vi "Find Worker Items.vi"(11 "Item Ref In":T1) -> (1 "Is Worker?":bool, 2 "Worker Items":T2, 3 "Item Ref":T1)   [LabVIEW 2020, in "FlexWorker_Provider.lvlib"]
uses:
  FlexWorker_Provider.lvlib
  <resource>/Framework/Providers/API/ItemRef.ctl
  Worker Items.ctl
  Worker Item.ctl
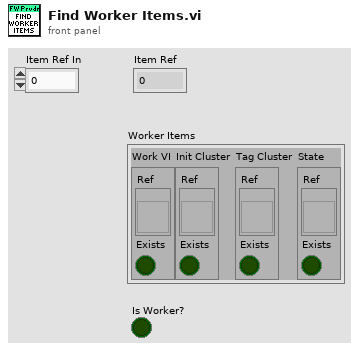
[diagram p1: front panel]
types:
  T1 = typedef "ItemRef.ctl" = u64
  T2 = typedef "FlexWorker_Provider.lvlib/Worker Items.ctl" = cluster{"Work VI":T3, "Init Cluster":T3, "Tag Cluster":T3, "State":T3}
  T3 = typedef "FlexWorker_Provider.lvlib/Worker Item.ctl" = cluster{"Ref":refnum<vi>, "Exists":bool}
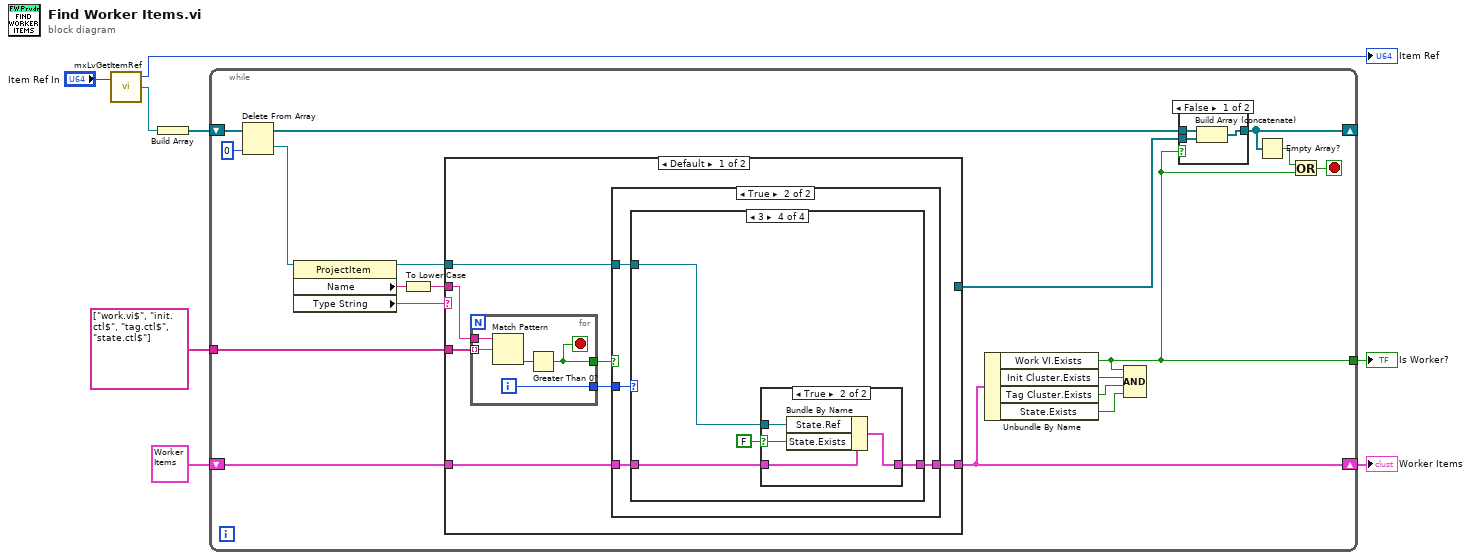
[diagram p0: block diagram]
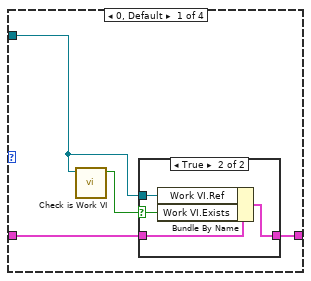
[diagram p4: hidden frame]
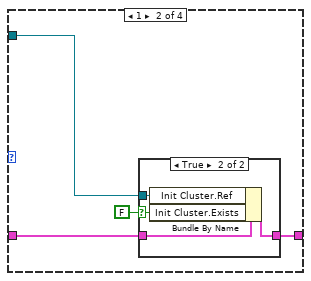
[diagram p6: hidden frame]
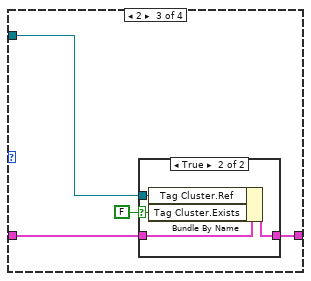
[diagram p8: hidden frame]
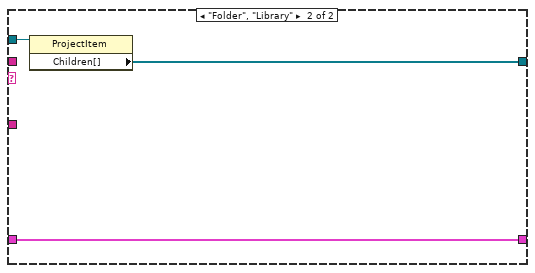
[diagram p11: hidden frame]
diagram:
  n1 = call <resource>:"mxLvGetItemRef.vi"("Item"="Item Ref In") -> ("Item"=→"Item Ref":T1, "Item Refnum"=w8:refnum<vi>)  [unwired: 1 in, 1 out]
  n2 = Build Array(w8) -> (w6:refnum<vi>[])
  n3 = while {
    shift-right: [w18] -> _
    shift-left: w6 -> [w27]
    shift-right: [w10] -> w4
    shift-left: T2 {"Work VI"={"Ref"=refnum, "Exists"=FALSE}, "Init Cluster"={"Ref"=refnum, "Exists"=FALSE}, "Tag Cluster"={"Ref"=refnum, "Exists"=FALSE}, "State"={"Ref"=refnum, "Exists"=FALSE}} ("Worker Items") -> [w20]
    tunnel: [w9] -> w3
    tunnel: string[] ["work.vi$", "init.ctl$", "tag.ctl$", "state.ctl$"] -> [w11]
    stop <- w15 stop-if-true
    n4 = Delete From Array(array=w27, index=0) -> (deleted portion=w25:refnum<vi>, array with subset deleted=w17:refnum<vi>[])  [unwired: 1 in]
    n5 = property class="ProjectItem"(reference=w25) -> (reference out=w23:refnum<vi>, "Name"=w24:string, "Type String"=w21:string)  [unwired: 1 in, 1 out]
    n6 = To Lower Case(string=w24) -> (all lower case string=w22:string)
    n7 = case shown="Default" w21 {
      tunnel: w23 -> [w34 w87]
      tunnel: w22 -> [w38 _]
      tunnel: w20 -> [w33 w85]
      tunnel: [_ w86] -> w16
      tunnel: [w32 w85] -> w10
      tunnel: w11 -> [w37 _]
      frame Default {
        n8 = for {
          tunnel: w38 -> [w84]
          tunnel: w37 -> [w83] mode=indexing
          tunnel: [w82] -> w35
          tunnel: [w80] -> w36
          i -> [w82]
          stop <- w80 stop-if-true
          n9 = Match Pattern(string=w84, regular expression=w83) -> (offset past match=w81:i32)  [unwired: 1 in, 3 out]
          n10 = Greater Than 0?(x=w81) -> (x > 0?=w80:bool)
        }
        n11 = case shown="True" w36 {
          tunnel: w35 -> [_ w42]
          tunnel: w34 -> [_ w43]
          tunnel: w33 -> [w39 w41]
          tunnel: [w39 w40] -> w32
          frame False {
            # "Not an item of interest"
          }
          frame True {
            n12 = case shown="3" w42 {
              tunnel: w43 -> [w44 w54 w63 w72]
              tunnel: w41 -> [w47 w56 w65 w74]
              tunnel: [w46 w55 w64 w73] -> w40
              frame 0, Default {
                n13 = call "Check is Work VI.vi"("Item Refnum"=w44) -> ("Work VI?"=w45:bool)  [unwired: 10 in]
                n14 = case shown="True" w45 {
                  selector: w45 -> [_ w51]
                  tunnel: w47 -> [w48 w52]
                  tunnel: [w48 w50] -> w46
                  tunnel: w44 -> [_ w49]
                  frame False {
                  }
                  frame True {
                    n15 = Bundle By Name(cluster=w52, "Work VI.Ref"=w49, "Work VI.Exists"=w51) -> (w50:T2)
                  }
                }
              }
              frame 1 {
                n16 = case shown="True" FALSE {
                  selector: FALSE -> [_ w60]
                  tunnel: w56 -> [w57 w61]
                  tunnel: [w57 w59] -> w55
                  tunnel: w54 -> [_ w58]
                  frame False {
                  }
                  frame True {
                    n17 = Bundle By Name(cluster=w61, "Init Cluster.Ref"=w58, "Init Cluster.Exists"=w60) -> (w59:T2)
                  }
                }
              }
              frame 2 {
                n18 = case shown="True" FALSE {
                  selector: FALSE -> [_ w69]
                  tunnel: w65 -> [w66 w70]
                  tunnel: [w66 w68] -> w64
                  tunnel: w63 -> [_ w67]
                  frame False {
                  }
                  frame True {
                    n19 = Bundle By Name(cluster=w70, "Tag Cluster.Ref"=w67, "Tag Cluster.Exists"=w69) -> (w68:T2)
                  }
                }
              }
              frame 3 {
                n20 = case shown="True" FALSE {
                  selector: FALSE -> [_ w78]
                  tunnel: w74 -> [w75 w79]
                  tunnel: [w75 w77] -> w73
                  tunnel: w72 -> [_ w76]
                  frame False {
                  }
                  frame True {
                    n21 = Bundle By Name(cluster=w79, "State.Ref"=w76, "State.Exists"=w78) -> (w77:T2)
                  }
                }
              }
            }
          }
        }
      }
      frame "Folder", "Library" {
        n22 = property class="ProjectItem"(reference=w87) -> ("Children[]"=w86:refnum<vi>[])  [unwired: 1 in, 2 out]
      }
    }
    n23 = Unbundle By Name(w10) -> ("Work VI.Exists"=w9:bool, "Init Cluster.Exists"=w14:bool, "Tag Cluster.Exists"=w13:bool, "State.Exists"=w12:bool)
    n24 = Compound Arithmetic op=AND(w9, w14, w13, w12) -> ()  [unwired: 1 out]
    n25 = case shown="False" w9 {
      tunnel: w17 -> [w30 w31]
      tunnel: w16 -> [w29 _]
      tunnel: [w28 w31] -> w18
      frame False {
        n26 = Build Array (concatenate)(w30, w29) -> (w28:refnum<vi>[])
      }
      frame True {
      }
    }
    n27 = Empty Array?(array=w18) -> (empty?=w19:bool)
    n28 = Or(x=w19, y=w9) -> (x .or. y?=w15:bool)
  }
  "Worker Items" <- w4
  "Is Worker?" <- w3
